vi "Test Set TDMS Property.vi"() -> ()   [LabVIEW 2015, in "Exposure Process.lvlib"]
uses:
  Exposure Process.lvlib
panel:
  in  "path":path
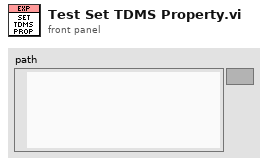
[diagram p1: front panel]
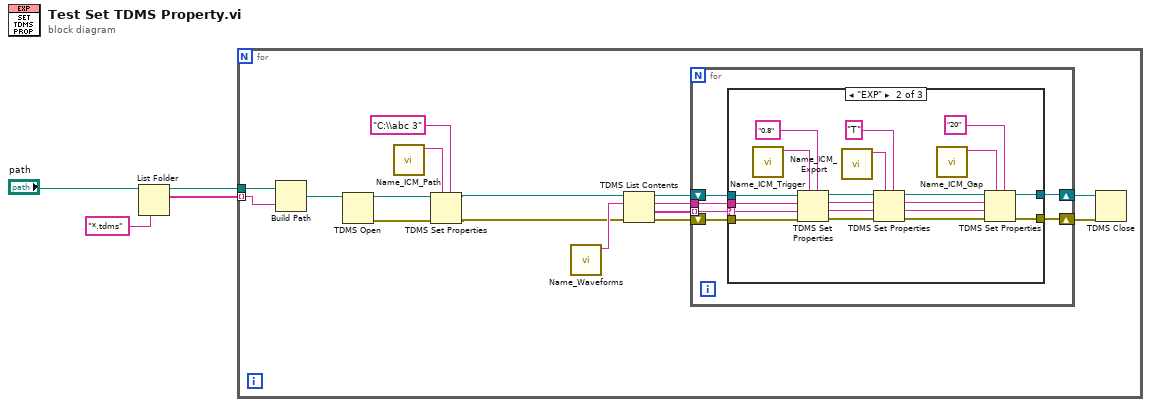
[diagram p0: block diagram]
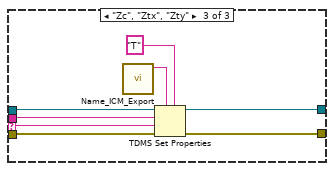
[diagram p3: hidden frame]
diagram:
  n1 = List Folder(path="path", pattern="*.tdms") -> (path out=w2:path, filenames=w1:string[])  [unwired: 2 in, 2 out]
  n2 = for {
    tunnel: w2 -> [w20]
    tunnel: w1 -> [w19] mode=indexing
    n3 = Build Path(base path=w20, name or relative path=w19) -> (appended path=w18:path)
    n4 = TDMS Open(11:w18) -> (0:w16:errorcluster, 3:w17:refnum<k34>)  [unwired: 6 in]
    n5 = call "Name_ICM_Path.vi"() -> ("Name"=w15:string)  [unwired: 11 in]
    n6 = TDMS Set Properties(5:"C:\\abc 3", 7:w15, 8:w16, 11:w17) -> (0:w5:errorcluster, 3:w6:refnum<k34>)  [unwired: 2 in, 2 out]
    n7 = call "Name_Waveforms.vi"() -> ("Name"=w13:string)  [unwired: 11 in]
    n8 = TDMS List Contents(4:w5, 6:w13, 7:w6) -> (0:w11:errorcluster, 1:w9:string[], 2:w10:string, 3:w12:refnum<k34>)
    n9 = for {
      tunnel: w10 -> [w23]
      tunnel: w9 -> [w25] mode=indexing
      shift-right: [w22] -> w7
      shift-left: w12 -> [w26]
      shift-right: [w21] -> w8
      shift-left: w11 -> [w24]
      n10 = case shown="\"EXP\"" w25 {
        selector: w25 -> [_ w45 w50]
        tunnel: w26 -> [w28 w48 w52]
        tunnel: w24 -> [w27 w47 w49]
        tunnel: w23 -> [_ w46 w51]
        tunnel: [w28 w31 w54] -> w22
        tunnel: [w27 w34 w53] -> w21
        frame Default {
        }
        frame "EXP" {
          n11 = call "Name_ICM_Trigger.vi"() -> ("Name"=w44:string)  [unwired: 11 in]
          n12 = TDMS Set Properties(5:"0.8", 7:w44, 8:w47, 9:w45, 10:w46, 11:w48) -> (0:w39:errorcluster, 1:w40:string, 2:w41:string, 3:w42:refnum<k34>)
          n13 = call "Name_ICM_Export.vi"() -> ("Name"=w38:string)  [unwired: 11 in]
          n14 = TDMS Set Properties(5:"T", 7:w38, 8:w39, 9:w40, 10:w41, 11:w42) -> (0:w32:errorcluster, 1:w29:string, 2:w30:string, 3:w33:refnum<k34>)
          n15 = call "Name_ICM_Gap.vi"() -> ("Name"=w35:string)  [unwired: 11 in]
          n16 = TDMS Set Properties(5:"20", 7:w35, 8:w32, 9:w29, 10:w30, 11:w33) -> (0:w34:errorcluster, 3:w31:refnum<k34>)  [unwired: 2 out]
        }
        frame "Zc", "Ztx", "Zty" {
          n17 = call "Name_ICM_Export.vi"() -> ("Name"=w56:string)  [unwired: 11 in]
          n18 = TDMS Set Properties(5:"T", 7:w56, 8:w49, 9:w50, 10:w51, 11:w52) -> (0:w53:errorcluster, 3:w54:refnum<k34>)  [unwired: 2 out]
        }
      }
    }
    n19 = TDMS Close(8:w8, 11:w7) -> ()  [unwired: 2 out]
  }
